vi "Handle Last Ack.vi"(8 "error in (no error)":errorcluster, 10 "Last Ack":refnum<class "Last Ack.lvclass">, 11 "Mediated Asynchronous Actor in":refnum<class "Mediated Asynchronous Actor.lvclass">) -> (0 "error out":errorcluster, 3 "Mediated Asynchronous Actor out":refnum<class "Mediated Asynchronous Actor.lvclass">)   [LabVIEW 2016, in "Stream Mediator.lvlib" / "Mediated Asynchronous Actor.lvclass"]
doc: "--\nCopyright © 2017 Composed SystemsI All rights reserved.\n\nAuthor: Jon McBee <jon.mcbee@composed.io>\n\nThis library is provided \"AS IS\" ,WITHOUT WARRANTIES OR\nCONDITIONS OF ANY KIND, either express or implied.\n\nComposed Systems -- composed.io\n\nStream 0.0.1.1\nJon McBee - Composed Systems\nCopyright (c) 2017, Composed Systems"
uses:
  <userlib>/Composed Systems/Stream/Mediator/Classes/Mediated Asynchronous Actor/Mediated Asynchronous Actor.lvclass
  <userlib>/Composed Systems/Stream/Mediator/Classes/Message Command Last Ack/Last Ack.lvclass
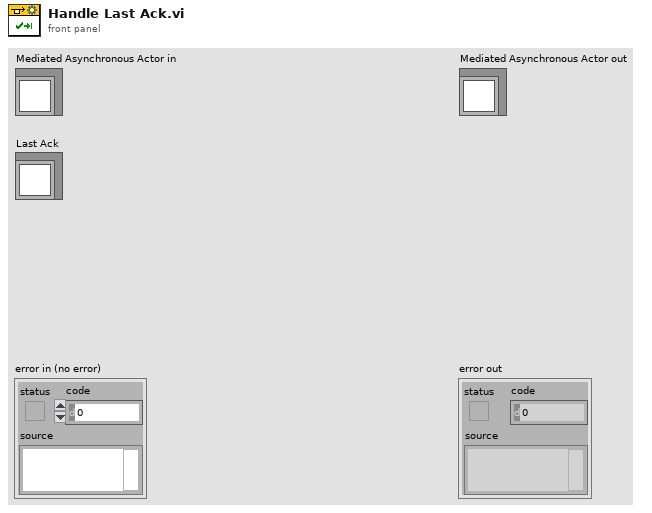
[diagram p1: front panel]
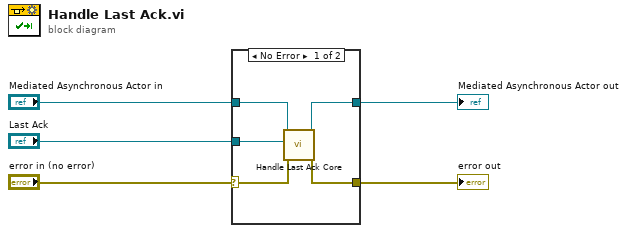
[diagram p0: block diagram]
diagram:
  n1 = case shown="No Error" "error in (no error)" {
    selector: "error in (no error)" -> [w7 w12]
    tunnel: [w6 w12] -> w4
    tunnel: [w9 w11] -> w2
    tunnel: "Mediated Asynchronous Actor in" -> [w10 w11]
    tunnel: "Last Ack" -> [w8 _]
    frame No Error {
      n2 = call-dynamic "Handle Last Ack Core.vi"("error in (no error)"=w7, "Last Ack"=w8, "Mediated Asynchronous Actor in"=w10) -> ("error out"=w6:errorcluster, "Mediated Asynchronous Actor out"=w9:refnum<class "Mediated Asynchronous Actor.lvclass">)  [unwired: 7 in]
    }
    frame Error {
    }
  }
  "error out" <- w4
  "Mediated Asynchronous Actor out" <- w2
